vi "PreProcess.vi"(8 "error in (no error)":errorcluster, 10 "Variant in":variant, 11 "ONNX EfficientNet Class in":refnum<class "ONNX EfficientNet Class.lvclass">) -> (0 "error out":errorcluster, 2 "Variant out":variant, 3 "ONNX EfficientNet Class out":refnum<class "ONNX EfficientNet Class.lvclass">)   [LabVIEW 2017, in "ONNX EfficientNet Class Library.lvlib" / "ONNX EfficientNet Class.lvclass"]
uses:
  ONNX EfficientNet Class.lvclass
  ONNX Angle Class/ONNX Angle Class Library.lvlib
  <vilib>/picture/picture.llb/imagedata.ctl
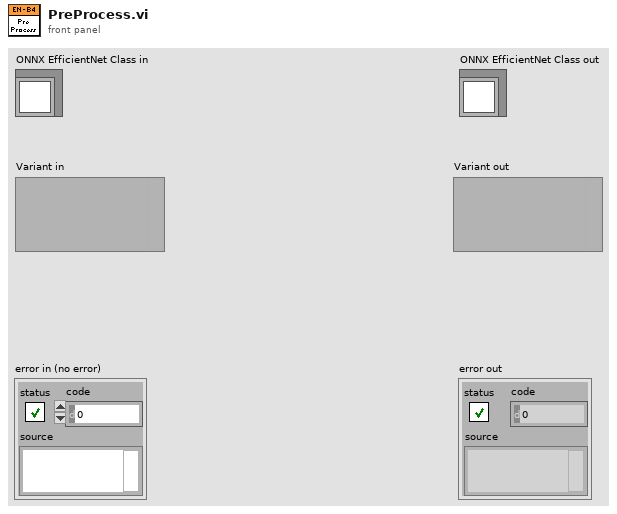
[diagram p1: front panel]
types:
  T1 = typedef "imagedata.ctl" = cluster{"image type":i32, "image depth":i32, "image":u8[], "mask":u8[], "colors":u32[], "Rectangle":cluster{"left":i16, "top":i16, "right":i16, "bottom":i16}}
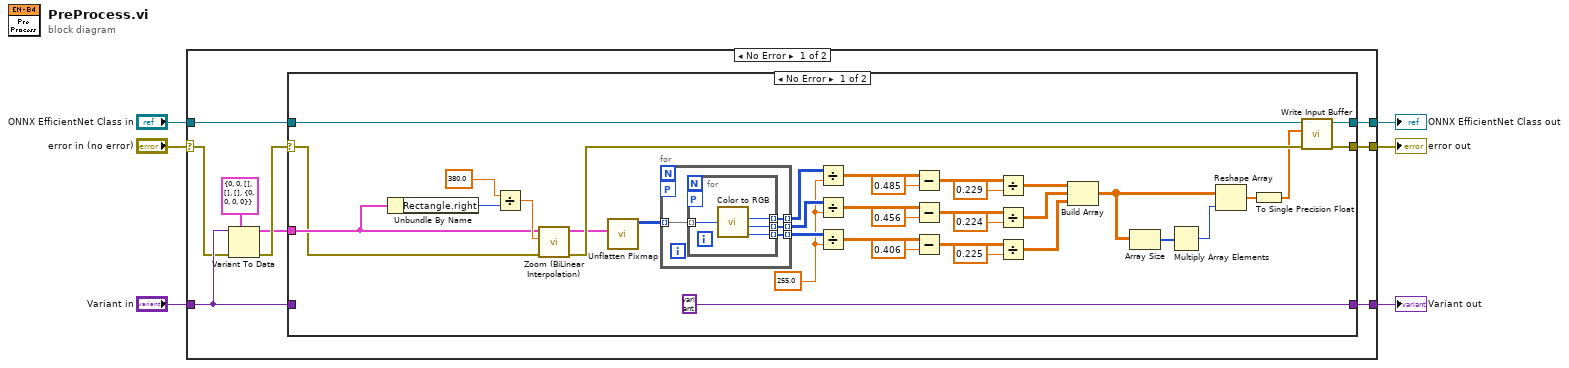
[diagram p0: block diagram]
diagram:
  n1 = case shown="No Error" "error in (no error)" {
    selector: "error in (no error)" -> [w9 w64]
    tunnel: "ONNX EfficientNet Class in" -> [w14 w65]
    tunnel: [w13 w65] -> w3
    tunnel: [w12 w64] -> w2
    tunnel: "Variant in" -> [w11 w63]
    tunnel: [w10 w63] -> w1
    frame No Error {
      n2 = Variant To Data(error in=w9, type=T1 {"image type"=0, "image depth"=0, "image"=[], "mask"=[], "colors"=[], "Rectangle"={"left"=0, "top"=0, "right"=0, "bottom"=0}} ("image data"), Variant=w11) -> (data=w8:T1, error out=w15:errorcluster)
      n3 = case shown="No Error" w15 {
        selector: w15 -> [w17 w61]
        tunnel: w8 -> [w18 _]
        tunnel: w14 -> [w51 w62]
        tunnel: [w50 w62] -> w13
        tunnel: [w49 w61] -> w12
        tunnel: w11 -> [_ w60]
        tunnel: [variant ("Variant in") w60] -> w10
        frame No Error {
          w36 = 255.0 ("y")
          n4 = Unbundle By Name(w18) -> ("Rectangle.right"=w48:i16)
          n5 = Divide(x=380.0, y=w48) -> (x/y=w47:dbl)
          n6 = call "Zoom (BiLinear Interpolation).vi"("error IN"=w17, "Zoom Coefficient"=w47, "image data IN"=w18) -> ("error OUT"=w45:errorcluster, "image data OUT"=w20:T1)  [unwired: 7 in]
          n7 = call <vilib>:"Unflatten Pixmap.vi"("image data"=w20) -> ("24-bit pixmap"=w44:u32[][])  [unwired: 10 out]
          n8 = for {
            tunnel: w44 -> [w55] mode=indexing
            tunnel: [w54] -> w37 mode=indexing
            tunnel: [w53] -> w38 mode=indexing
            tunnel: [w52] -> w39 mode=indexing
            workers-P: _ -> [_]
            n9 = for {
              tunnel: w55 -> [w56] mode=indexing
              tunnel: [w59] -> w54 mode=indexing
              tunnel: [w58] -> w53 mode=indexing
              tunnel: [w57] -> w52 mode=indexing
              workers-P: _ -> [_]
              n10 = call <vilib>:"Color to RGB.vi"("Color"=w56) -> ("R"=w59:u8, "G"=w58:u8, "B"=w57:u8)  [unwired: 1 out]
            }
          }
          n11 = Divide(x=w37, y=w36) -> (x/y=w35:dbl[][])
          n12 = Divide(x=w38, y=w36) -> (x/y=w24:dbl[][])
          n13 = Divide(x=w39, y=w36) -> (x/y=w22:dbl[][])
          n14 = Subtract(x=w35, y=0.485) -> (x-y=w33:dbl[][])
          n15 = Subtract(x=w24, y=0.456) -> (x-y=w25:dbl[][])
          n16 = Subtract(x=w22, y=0.406) -> (x-y=w27:dbl[][])
          n17 = Divide(x=w33, y=0.229) -> (x/y=w32:dbl[][])
          n18 = Divide(x=w25, y=0.224) -> (x/y=w23:dbl[][])
          n19 = Divide(x=w27, y=0.225) -> (x/y=w21:dbl[][])
          n20 = Build Array(w32, w23, w21) -> (w41:dbl[][][])
          n21 = Array Size(array=w41) -> (size(s)=w40:i32[])
          n22 = Multiply Array Elements(1:w40) -> (0:w42:i32)
          n23 = Reshape Array(w41, w42) -> (w43:dbl[])
          n24 = To Single Precision Float(number=w43) -> (single precision float=w19:sgl[])
          n25 = call-dynamic "Write Input Buffer.vi"("error in (no error)"=w45, "Input Buffer"=w19, "ONNX Class in"=w51) -> ("error out"=w49:errorcluster, "ONNX Class out"=w50:refnum<class "ONNX EfficientNet Class.lvclass">)  [unwired: 7 in]
        }
        frame Error {
        }
      }
    }
    frame Error {
    }
  }
  "error out" <- w2
  "ONNX EfficientNet Class out" <- w3
  "Variant out" <- w1
